vi "AuMT8852B VI Tree.vi"   [LabVIEW 2017]
doc: "This is the instrument driver for the MT8852B. The VI Tree displays all the user-callable VIs of the instrument driver in an organized table."
panel:
  # "SEE DIAGRAM\nFOR VI TREE."
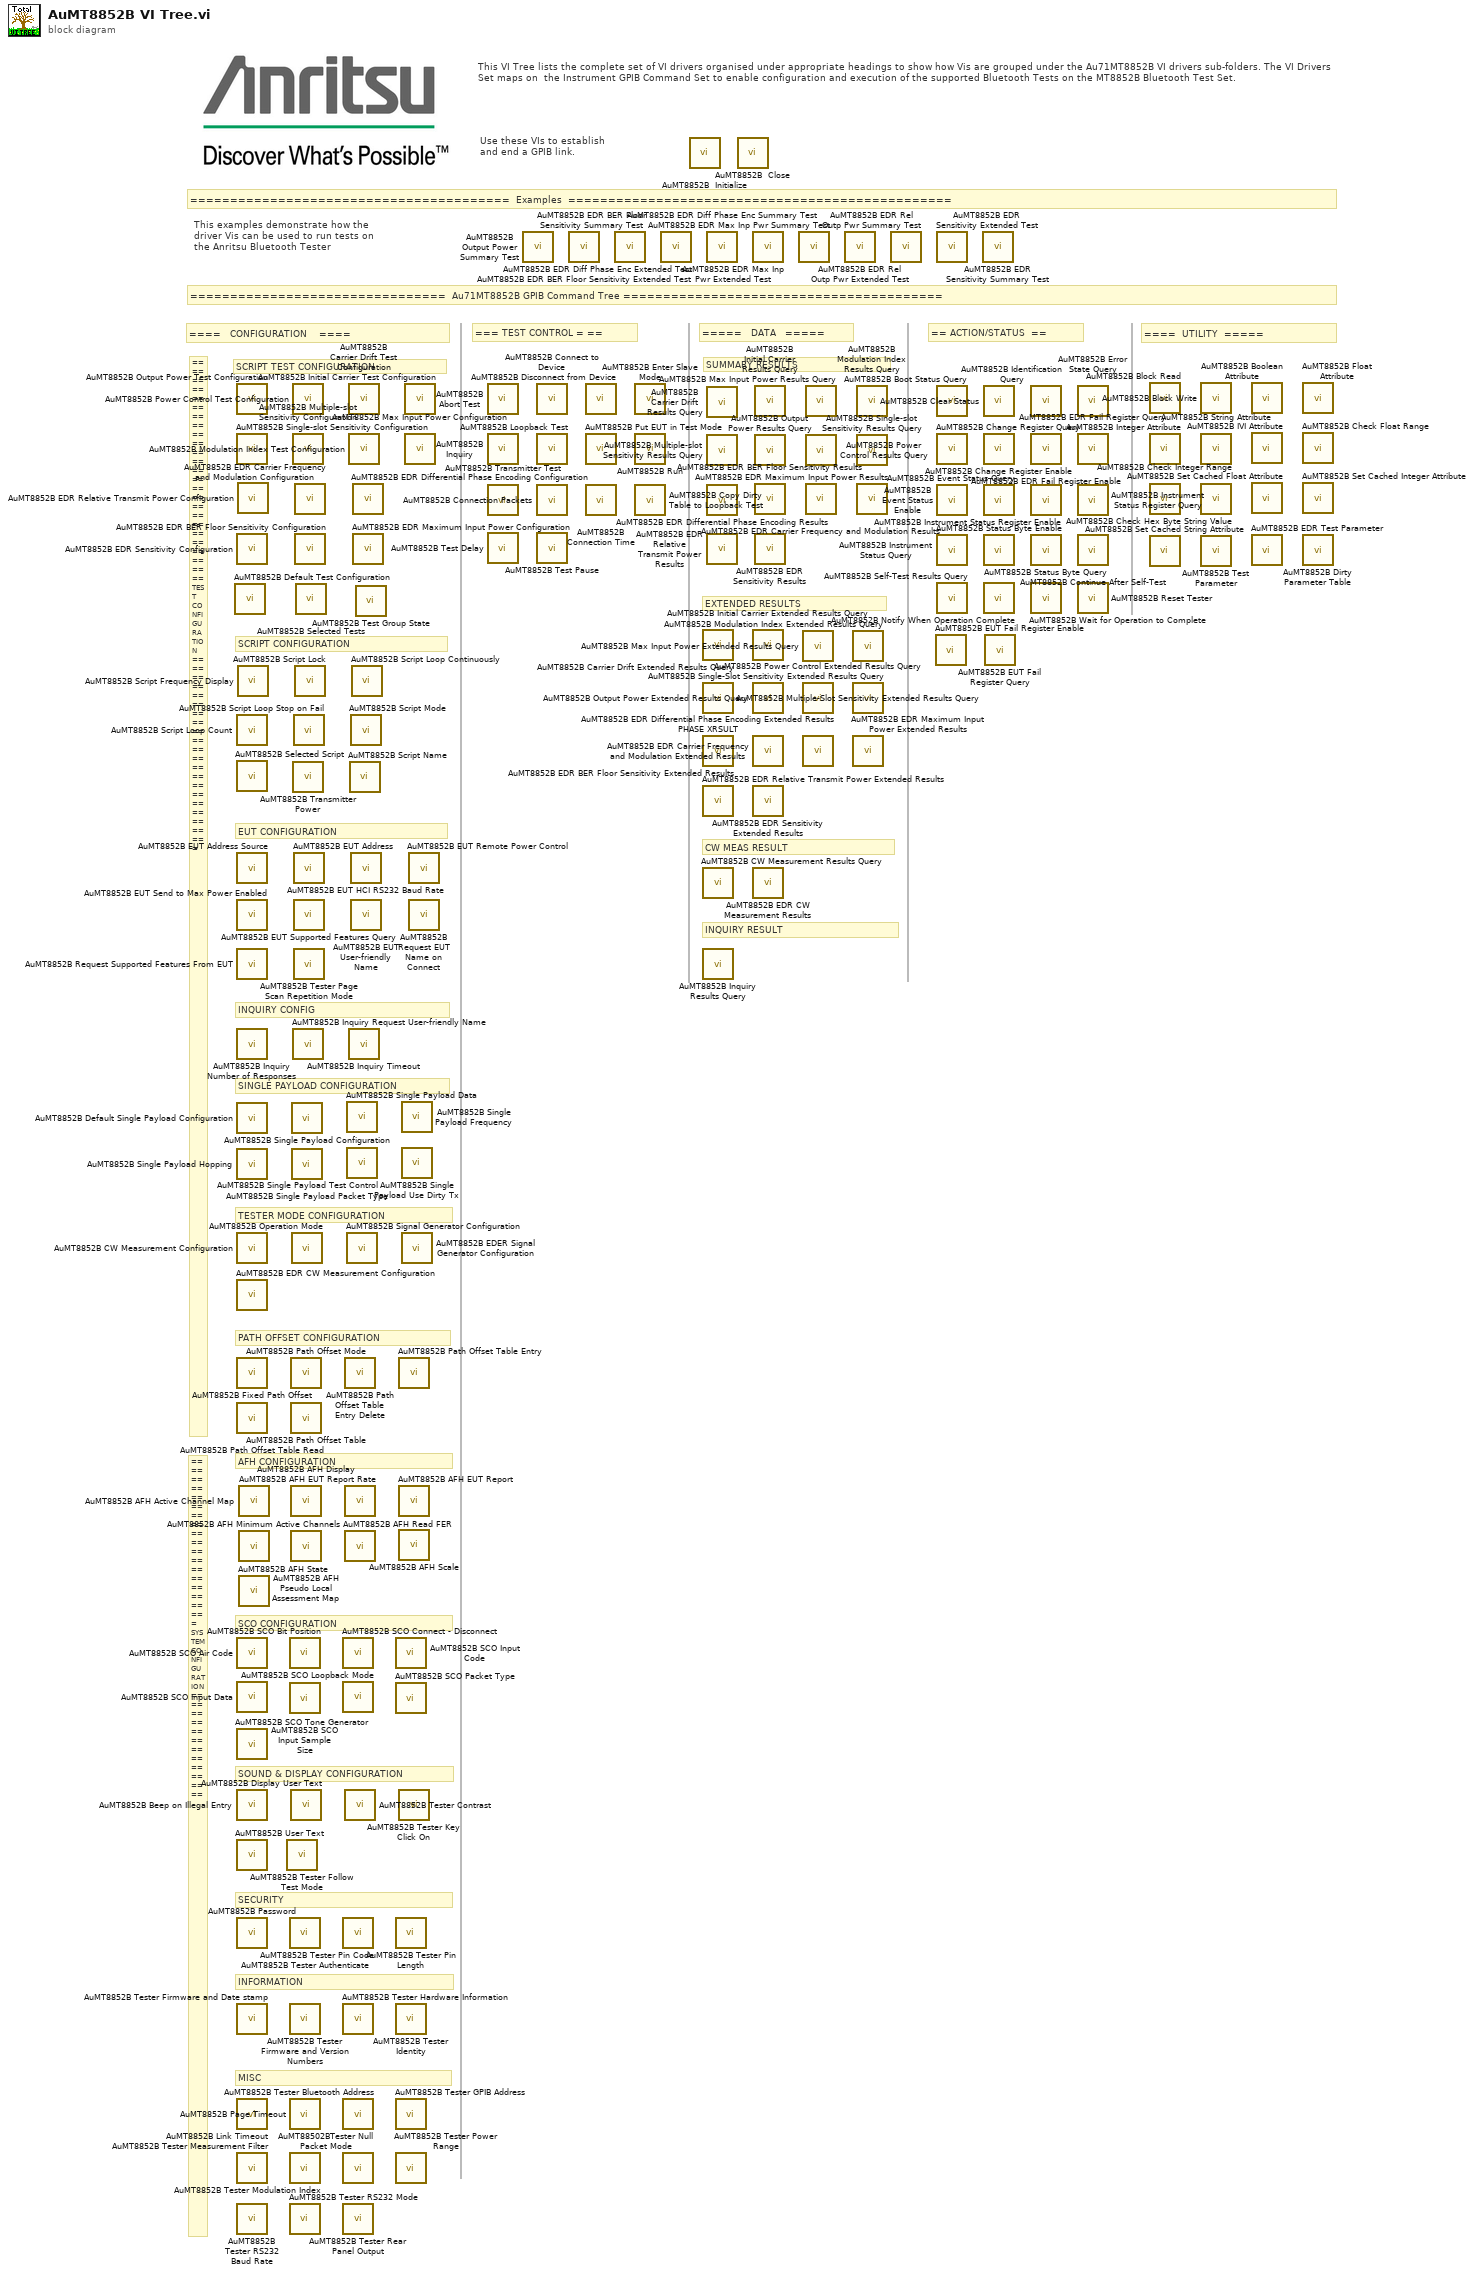
[diagram p0: block diagram]
diagram:
  # "This examples demonstrate how the \ndriver Vis can be used to run tests on \nthe Anritsu Bluetooth Tester"
  # "========================================  Examples  ================================================"
  # "=== TEST CONTROL = =="
  # "SCRIPT CONFIGURATION"
  # "===================================== SYSTEM CONFIGURATION ========================"
  # "INQUIRY RESULT"
  # "CW MEAS RESULT"
  # "EXTENDED RESULTS"
  # "SUMMARY RESULTS"
  # "MISC"
  # "INFORMATION"
  # "SECURITY"
  # "SOUND & DISPLAY CONFIGURATION"
  # "SCO CONFIGURATION"
  # "AFH CONFIGURATION"
  # "INQUIRY CONFIG"
  # "TESTER MODE CONFIGURATION"
  # "PATH OFFSET CONFIGURATION"
  # "EUT CONFIGURATION"
  # "SCRIPT TEST CONFIGURATION"
  # "SINGLE PAYLOAD CONFIGURATION"
  # "================================================== TEST CONFIGURATION ==========================================="
  # "====  UTILITY  ====="
  # "== ACTION/STATUS  =="
  # "=====   DATA   ====="
  # "This VI Tree lists the complete set of VI drivers organised under appropriate headings to show how Vis are grouped under the Au71MT8852B VI drivers sub-folders. The VI Drivers Set maps on  the Instrument GPIB Command Set to enable configuration and execution of the supported Bluetooth Tests on the MT8852B Bluetooth Test Set."
  # "Use these VIs to establish \nand end a GPIB link."
  # "====   CONFIGURATION    ===="
  # "================================  Au71MT8852B GPIB Command Tree ========================================"
  n1 = call <instrlib>:"AuMT8852B Default Test Configuration.vi"() -> ()  [unwired: 9 in, 3 out]
  n2 = call <instrlib>:"AuMT8852B Output Power Test Configuration.vi"() -> ()  [unwired: 8 in, 4 out]
  n3 = call <instrlib>:"AuMT8852B Single-slot Sensitivity Configuration.vi"() -> ()  [unwired: 8 in, 4 out]
  n4 = call <instrlib>:"AuMT8852B EDR Sensitivity Configuration.vi"() -> ()  [unwired: 8 in, 4 out]
  n5 = call <instrlib>:"AuMT8852B Script Loop Count.vi"() -> ()  [unwired: 8 in, 4 out]
  n6 = call <instrlib>:"AuMT8852B Selected Script.vi"() -> ()  [unwired: 8 in, 4 out]
  n7 = call <instrlib>:"AuMT8852B EUT Address Source.vi"() -> ()  [unwired: 8 in, 4 out]
  n8 = call <instrlib>:"AuMT8852B EUT Send to Max Power Enabled.vi"() -> ()  [unwired: 8 in, 4 out]
  n9 = call <instrlib>:"AuMT8852B Request Supported Features From EUT.vi"() -> ()  [unwired: 9 in, 3 out]
  n10 = call <instrlib>:"AuMT8852B Inquiry Number of Responses.vi"() -> ()  [unwired: 8 in, 4 out]
  n11 = call <instrlib>:"AuMT8852B Default Single Payload Configuration.vi"() -> ()  [unwired: 9 in, 3 out]
  n12 = call <instrlib>:"AuMT8852B Single Payload Hopping.vi"() -> ()  [unwired: 8 in, 4 out]
  n13 = call <instrlib>:"AuMT8852B CW Measurement Configuration.vi"() -> ()  [unwired: 6 in, 6 out]
  n14 = call <instrlib>:"AuMT8852B EDR CW Measurement Configuration.vi"() -> ()  [unwired: 8 in, 4 out]
  n15 = call <instrlib>:"AuMT8852B Fixed Path Offset.vi"() -> ()  [unwired: 8 in, 4 out]
  n16 = call <instrlib>:"AuMT8852B Path Offset Table Read.vi"() -> ()  [unwired: 8 in, 4 out]
  n17 = call <instrlib>:"AuMT8852B SCO Air Code.vi"() -> ()  [unwired: 8 in, 4 out]
  n18 = call <instrlib>:"AuMT8852B SCO Input Data.vi"() -> ()  [unwired: 8 in, 4 out]
  n19 = call <instrlib>:"AuMT8852B SCO Tone Generator.vi"() -> ()  [unwired: 8 in, 4 out]
  n20 = call <instrlib>:"AuMT8852B Beep on Illegal Entry.vi"() -> ()  [unwired: 8 in, 4 out]
  n21 = call <instrlib>:"AuMT8852B User Text.vi"() -> ()  [unwired: 8 in, 4 out]
  n22 = call <instrlib>:"AuMT8852B Password.vi"() -> ()  [unwired: 9 in, 3 out]
  n23 = call <instrlib>:"AuMT8852B Tester Firmware and Date stamp.vi"() -> ()  [unwired: 8 in, 4 out]
  n24 = call <instrlib>:"AuMT8852B Link Timeout.vi"() -> ()  [unwired: 8 in, 4 out]
  n25 = call <instrlib>:"AuMT8852B Tester Measurement Filter.vi"() -> ()  [unwired: 8 in, 4 out]
  n26 = call <instrlib>:"AuMT8852B Tester RS232 Baud Rate.vi"() -> ()  [unwired: 8 in, 4 out]
  n27 = call <instrlib>:"AuMT8852B EDR Relative Transmit Power Configuration.vi"() -> ()  [unwired: 8 in, 4 out]
  n28 = call <instrlib>:"AuMT8852B Script Frequency Display.vi"() -> ()  [unwired: 8 in, 4 out]
  n29 = call <instrlib>:"AuMT8852B AFH Active Channel Map.vi"() -> ()  [unwired: 7 in, 5 out]
  n30 = call <instrlib>:"AuMT8852B AFH Minimum Active Channels.vi"() -> ()  [unwired: 8 in, 4 out]
  n31 = call <instrlib>:"AuMT8852B AFH State.vi"() -> ()  [unwired: 8 in, 4 out]
  n32 = call <instrlib>:"AuMT8852B Tester Follow Test Mode.vi"() -> ()  [unwired: 8 in, 4 out]
  n33 = call <instrlib>:"AuMT8852B SCO Bit Position.vi"() -> ()  [unwired: 8 in, 4 out]
  n34 = call <instrlib>:"AuMT8852B SCO Input Sample Size.vi"() -> ()  [unwired: 8 in, 4 out]
  n35 = call <instrlib>:"AuMT8852B Tester Authenticate.vi"() -> ()  [unwired: 8 in, 4 out]
  n36 = call <instrlib>:"AuMT8852B Tester Firmware and Version Numbers.vi"() -> ()  [unwired: 8 in, 4 out]
  n37 = call <instrlib>:"AuMT8852B Page Timeout.vi"() -> ()  [unwired: 8 in, 4 out]
  n38 = call <instrlib>:"AuMT8852B Tester Modulation Index.vi"() -> ()  [unwired: 8 in, 4 out]
  n39 = call <instrlib>:"AuMT8852B Tester RS232 Mode.vi"() -> ()  [unwired: 8 in, 4 out]
  n40 = call <instrlib>:"AuMT8852B Path Offset Mode.vi"() -> ()  [unwired: 8 in, 4 out]
  n41 = call <instrlib>:"AuMT8852B Path Offset Table.vi"() -> ()  [unwired: 8 in, 4 out]
  n42 = call <instrlib>:"AuMT8852B AFH Display.vi"() -> ()  [unwired: 8 in, 4 out]
  n43 = call <instrlib>:"AuMT8852B AFH Pseudo Local Assessment Map.vi"() -> ()  [unwired: 9 in, 3 out]
  n44 = call <instrlib>:"AuMT8852B Display User Text.vi"() -> ()  [unwired: 8 in, 4 out]
  n45 = call <instrlib>:"AuMT8852B Single Payload Configuration.vi"() -> ()  [unwired: 8 in, 4 out]
  n46 = call <instrlib>:"AuMT8852B Single Payload Packet Type.vi"() -> ()  [unwired: 8 in, 4 out]
  n47 = call <instrlib>:"AuMT8852B Operation Mode.vi"() -> ()  [unwired: 8 in, 4 out]
  n48 = call <instrlib>:"AuMT8852B Power Control Test Configuration.vi"() -> ()  [unwired: 8 in, 4 out]
  n49 = call <instrlib>:"AuMT8852B Multiple-slot Sensitivity Configuration.vi"() -> ()  [unwired: 8 in, 4 out]
  n50 = call <instrlib>:"AuMT8852B Transmitter Power.vi"() -> ()  [unwired: 8 in, 4 out]
  n51 = call <instrlib>:"AuMT8852B Inquiry Request User-friendly Name.vi"() -> ()  [unwired: 8 in, 4 out]
  n52 = call <instrlib>:"AuMT8852B Script Loop Stop on Fail.vi"() -> ()  [unwired: 8 in, 4 out]
  n53 = call <instrlib>:"AuMT8852B EUT Address.vi"() -> ()  [unwired: 8 in, 4 out]
  n54 = call <instrlib>:"AuMT8852B EUT Supported Features Query.vi"() -> ()  [unwired: 8 in, 4 out]
  n55 = call <instrlib>:"AuMT8852B Tester Page Scan Repetition Mode.vi"() -> ()  [unwired: 8 in, 4 out]
  n56 = call <instrlib>:"AuMT8852B EDR Carrier Frequency and Modulation Configuration.vi"() -> ()  [unwired: 8 in, 4 out]
  n57 = call <instrlib>:"AuMT8852B EDR BER Floor Sensitivity Configuration.vi"() -> ()  [unwired: 8 in, 4 out]
  n58 = call <instrlib>:"AuMT8852B Script Lock.vi"() -> ()  [unwired: 8 in, 4 out]
  n59 = call <instrlib>:"AuMT8852B Selected Tests.vi"() -> ()  [unwired: 8 in, 4 out]
  n60 = call <instrlib>:"AuMT8852B SCO Connect - Disconnect.vi"() -> ()  [unwired: 9 in, 3 out]
  n61 = call <instrlib>:"AuMT8852B SCO Loopback Mode.vi"() -> ()  [unwired: 8 in, 4 out]
  n62 = call <instrlib>:"AuMT8852B Tester Pin Code.vi"() -> ()  [unwired: 8 in, 4 out]
  n63 = call <instrlib>:"AuMT8852B Tester Hardware Information.vi"() -> ()  [unwired: 8 in, 4 out]
  n64 = call <instrlib>:"AuMT8852B Tester Bluetooth Address.vi"() -> ()  [unwired: 8 in, 4 out]
  n65 = call <instrlib>:"AuMT88502BTester Null Packet Mode.vi"() -> ()  [unwired: 8 in, 4 out]
  n66 = call <instrlib>:"AuMT8852B Tester Rear Panel Output.vi"() -> ()  [unwired: 8 in, 4 out]
  n67 = call <instrlib>:"AuMT8852B Path Offset Table Entry Delete.vi"() -> ()  [unwired: 9 in, 3 out]
  n68 = call <instrlib>:"AuMT8852B AFH EUT Report Rate.vi"() -> ()  [unwired: 8 in, 4 out]
  n69 = call <instrlib>:"AuMT8852B AFH Read FER.vi"() -> ()  [unwired: 8 in, 4 out]
  n70 = call <instrlib>:"AuMT8852B Tester Contrast.vi"() -> ()  [unwired: 8 in, 4 out]
  n71 = call <instrlib>:"AuMT8852B Single Payload Data.vi"() -> ()  [unwired: 8 in, 4 out]
  n72 = call <instrlib>:"AuMT8852B Single Payload Test Control.vi"() -> ()  [unwired: 8 in, 4 out]
  n73 = call <instrlib>:"AuMT8852B Signal Generator Configuration.vi"() -> ()  [unwired: 8 in, 4 out]
  n74 = call <instrlib>:"AuMT8852B Carrier Drift Test Configuration.vi"() -> ()  [unwired: 8 in, 4 out]
  n75 = call <instrlib>:"AuMT8852B Modulation Index Test Configuration.vi"() -> ()  [unwired: 8 in, 4 out]
  n76 = call <instrlib>:"AuMT8852B Inquiry Timeout.vi"() -> ()  [unwired: 8 in, 4 out]
  n77 = call <instrlib>:"AuMT8852B Script Name.vi"() -> ()  [unwired: 8 in, 4 out]
  n78 = call <instrlib>:"AuMT8852B Script Mode.vi"() -> ()  [unwired: 8 in, 4 out]
  n79 = call <instrlib>:"AuMT8852B EUT HCI RS232 Baud Rate.vi"() -> ()  [unwired: 8 in, 4 out]
  n80 = call <instrlib>:"AuMT8852B EUT User-friendly Name.vi"() -> ()  [unwired: 8 in, 4 out]
  n81 = call <instrlib>:"AuMT8852B Script Loop Continuously.vi"() -> ()  [unwired: 8 in, 4 out]
  n82 = call <instrlib>:"AuMT8852B EDR Differential Phase Encoding Configuration.vi"() -> ()  [unwired: 8 in, 4 out]
  n83 = call <instrlib>:"AuMT8852B EDR Maximum Input Power Configuration.vi"() -> ()  [unwired: 8 in, 4 out]
  n84 = call <instrlib>:"AuMT8852B Test Group State.vi"() -> ()  [unwired: 7 in, 5 out]
  n85 = call <instrlib>:"AuMT8852B SCO Input Code.vi"() -> ()  [unwired: 8 in, 4 out]
  n86 = call <instrlib>:"AuMT8852B SCO Packet Type.vi"() -> ()  [unwired: 8 in, 4 out]
  n87 = call <instrlib>:"AuMT8852B Tester Pin Length.vi"() -> ()  [unwired: 8 in, 4 out]
  n88 = call <instrlib>:"AuMT8852B Tester Identity.vi"() -> ()  [unwired: 8 in, 4 out]
  n89 = call <instrlib>:"AuMT8852B Tester GPIB Address.vi"() -> ()  [unwired: 8 in, 4 out]
  n90 = call <instrlib>:"AuMT8852B Tester Power Range.vi"() -> ()  [unwired: 8 in, 4 out]
  n91 = call <instrlib>:"AuMT8852B Path Offset Table Entry.vi"() -> ()  [unwired: 8 in, 4 out]
  n92 = call <instrlib>:"AuMT8852B AFH EUT Report.vi"() -> ()  [unwired: 8 in, 4 out]
  n93 = call <instrlib>:"AuMT8852B AFH Scale.vi"() -> ()  [unwired: 8 in, 4 out]
  n94 = call <instrlib>:"AuMT8852B Tester Key Click On.vi"() -> ()  [unwired: 8 in, 4 out]
  n95 = call <instrlib>:"AuMT8852B Single Payload Frequency.vi"() -> ()  [unwired: 8 in, 4 out]
  n96 = call <instrlib>:"AuMT8852B Single Payload Use Dirty Tx.vi"() -> ()  [unwired: 8 in, 4 out]
  n97 = call <instrlib>:"AuMT8852B EDER Signal Generator Configuration.vi"() -> ()  [unwired: 8 in, 4 out]
  n98 = call <instrlib>:"AuMT8852B Initial Carrier Test Configuration.vi"() -> ()  [unwired: 8 in, 4 out]
  n99 = call <instrlib>:"AuMT8852B Max Input Power Configuration.vi"() -> ()  [unwired: 8 in, 4 out]
  n100 = call <instrlib>:"AuMT8852B EUT Remote Power Control.vi"() -> ()  [unwired: 9 in, 3 out]
  n101 = call <instrlib>:"AuMT8852B Request EUT Name on Connect.vi"() -> ()  [unwired: 8 in, 4 out]
  n102 = call <instrlib>:"AuMT8852B Abort Test.vi"() -> ()  [unwired: 9 in, 3 out]
  n103 = call <instrlib>:"AuMT8852B Inquiry.vi"() -> ()  [unwired: 9 in, 3 out]
  n104 = call <instrlib>:"AuMT8852B Transmitter Test.vi"() -> ()  [unwired: 9 in, 3 out]
  n105 = call <instrlib>:"AuMT8852B Test Delay.vi"() -> ()  [unwired: 8 in, 4 out]
  n106 = call <instrlib>:"AuMT8852B Output Power Summary Test.vi"() -> ()  [unwired: 1 in]
  n107 = call <instrlib>:"AuMT8852B Connect to Device.vi"() -> ()  [unwired: 9 in, 3 out]
  n108 = call <instrlib>:"AuMT8852B Loopback Test.vi"() -> ()  [unwired: 9 in, 3 out]
  n109 = call <instrlib>:"AuMT8852B Connection Packets.vi"() -> ()  [unwired: 8 in, 4 out]
  n110 = call <instrlib>:"AuMT8852B Test Pause.vi"() -> ()  [unwired: 8 in, 4 out]
  n111 = call <instrlib>:"AuMT8852B EDR BER Floor Sensitivity Extended Test.vi"() -> ()  [unwired: 1 in]
  n112 = call <instrlib>:"AuMT8852B Disconnect from Device.vi"() -> ()  [unwired: 9 in, 3 out]
  n113 = call <instrlib>:"AuMT8852B Put EUT in Test Mode.vi"() -> ()  [unwired: 9 in, 3 out]
  n114 = call <instrlib>:"AuMT8852B Connection Time.vi"() -> ()  [unwired: 8 in, 4 out]
  n115 = call <instrlib>:"AuMT8852B EDR BER Floor Sensitivity Summary Test.vi"() -> ()  [unwired: 1 in]
  n116 = call <instrlib>:"AuMT8852B Enter Slave Mode.vi"() -> ()  [unwired: 9 in, 3 out]
  n117 = call <instrlib>:"AuMT8852B Run.vi"() -> ()  [unwired: 9 in, 3 out]
  n118 = call <instrlib>:"AuMT8852B Copy Dirty Table to Loopback Test.vi"() -> ()  [unwired: 9 in, 3 out]
  n119 = call <instrlib>:"AuMT8852B EDR Diff Phase Enc Extended Test.vi"() -> ()  [unwired: 1 in]
  n120 = call <instrlib>:"AuMT8852B  Initialize.vi"() -> ()  [unwired: 10 in, 2 out]
  n121 = call <instrlib>:"AuMT8852B Carrier Drift Extended Results Query.vi"() -> ()  [unwired: 8 in, 4 out]
  n122 = call <instrlib>:"AuMT8852B Multiple-Slot Sensitivity Extended Results Query.vi"() -> ()  [unwired: 8 in, 4 out]
  n123 = call <instrlib>:"AuMT8852B EDR BER Floor Sensitivity Extended Results.vi"() -> ()  [unwired: 8 in, 4 out]
  n124 = call <instrlib>:"AuMT8852B EDR Relative Transmit Power Extended Results.vi"() -> ()  [unwired: 8 in, 4 out]
  n125 = call <instrlib>:"AuMT8852B CW Measurement Results Query.vi"() -> ()  [unwired: 8 in, 4 out]
  n126 = call <instrlib>:"AuMT8852B Inquiry Results Query.vi"() -> ()  [unwired: 7 in, 5 out]
  n127 = call <instrlib>:"AuMT8852B EDR Diff Phase Enc Summary Test.vi"() -> ()  [unwired: 1 in]
  n128 = call <instrlib>:"AuMT8852B Carrier Drift Results Query.vi"() -> ()  [unwired: 8 in, 4 out]
  n129 = call <instrlib>:"AuMT8852B Multiple-slot Sensitivity Results Query.vi"() -> ()  [unwired: 8 in, 4 out]
  n130 = call <instrlib>:"AuMT8852B EDR Differential Phase Encoding Results.vi"() -> ()  [unwired: 8 in, 4 out]
  n131 = call <instrlib>:"AuMT8852B EDR Relative Transmit Power Results.vi"() -> ()  [unwired: 8 in, 4 out]
  n132 = call <instrlib>:"AuMT8852B  Close.vi"() -> ()  [unwired: 10 in, 2 out]
  n133 = call <instrlib>:"AuMT8852B EDR Max Inp Pwr Extended Test.vi"() -> ()  [unwired: 1 in]
  n134 = call <instrlib>:"AuMT8852B Initial Carrier Extended Results Query.vi"() -> ()  [unwired: 8 in, 4 out]
  n135 = call <instrlib>:"AuMT8852B Output Power Extended Results Query.vi"() -> ()  [unwired: 8 in, 4 out]
  n136 = call <instrlib>:"AuMT8852B EDR Carrier Frequency and Modulation Extended Results.vi"() -> ()  [unwired: 8 in, 4 out]
  n137 = call <instrlib>:"AuMT8852B EDR Sensitivity Extended Results.vi"() -> ()  [unwired: 8 in, 4 out]
  n138 = call <instrlib>:"AuMT8852B EDR CW Measurement Results.vi"() -> ()  [unwired: 8 in, 4 out]
  n139 = call <instrlib>:"AuMT8852B Initial Carrier Results Query.vi"() -> ()  [unwired: 8 in, 4 out]
  n140 = call <instrlib>:"AuMT8852B Output Power Results Query.vi"() -> ()  [unwired: 8 in, 4 out]
  n141 = call <instrlib>:"AuMT8852B EDR BER Floor Sensitivity Results.vi"() -> ()  [unwired: 8 in, 4 out]
  n142 = call <instrlib>:"AuMT8852B EDR Sensitivity Results.vi"() -> ()  [unwired: 8 in, 4 out]
  n143 = call <instrlib>:"AuMT8852B EDR Max Inp Pwr Summary Test.vi"() -> ()  [unwired: 1 in]
  n144 = call <instrlib>:"AuMT8852B Max Input Power Extended Results Query.vi"() -> ()  [unwired: 8 in, 4 out]
  n145 = call <instrlib>:"AuMT8852B Power Control Extended Results Query.vi"() -> ()  [unwired: 8 in, 4 out]
  n146 = call <instrlib>:"AuMT8852B EDR Differential Phase Encoding Extended Results PHASE XRSULT.vi"() -> ()  [unwired: 8 in, 4 out]
  n147 = call <instrlib>:"AuMT8852B Max Input Power Results Query.vi"() -> ()  [unwired: 8 in, 4 out]
  n148 = call <instrlib>:"AuMT8852B Power Control Results Query.vi"() -> ()  [unwired: 8 in, 4 out]
  n149 = call <instrlib>:"AuMT8852B EDR Carrier Frequency and Modulation Results.vi"() -> ()  [unwired: 8 in, 4 out]
  n150 = call <instrlib>:"AuMT8852B EDR Rel Outp Pwr Extended Test.vi"() -> ()  [unwired: 1 in]
  n151 = call <instrlib>:"AuMT8852B Modulation Index Extended Results Query.vi"() -> ()  [unwired: 8 in, 4 out]
  n152 = call <instrlib>:"AuMT8852B Single-Slot Sensitivity Extended Results Query.vi"() -> ()  [unwired: 8 in, 4 out]
  n153 = call <instrlib>:"AuMT8852B EDR Maximum Input Power Extended Results.vi"() -> ()  [unwired: 8 in, 4 out]
  n154 = call <instrlib>:"AuMT8852B Modulation Index Results Query.vi"() -> ()  [unwired: 8 in, 4 out]
  n155 = call <instrlib>:"AuMT8852B Single-slot Sensitivity Results Query.vi"() -> ()  [unwired: 8 in, 4 out]
  n156 = call <instrlib>:"AuMT8852B EDR Maximum Input Power Results.vi"() -> ()  [unwired: 8 in, 4 out]
  n157 = call <instrlib>:"AuMT8852B EDR Rel Outp Pwr Summary Test.vi"() -> ()  [unwired: 1 in]
  n158 = call <instrlib>:"AuMT8852B EUT Fail Register Enable.vi"() -> ()  [unwired: 7 in, 5 out]
  n159 = call <instrlib>:"AuMT8852B EDR Sensitivity Extended Test.vi"() -> ()  [unwired: 1 in]
  n160 = call <instrlib>:"AuMT8852B Boot Status Query.vi"() -> ()  [unwired: 8 in, 4 out]
  n161 = call <instrlib>:"AuMT8852B Change Register Query.vi"() -> ()  [unwired: 7 in, 5 out]
  n162 = call <instrlib>:"AuMT8852B Event Status Enable.vi"() -> ()  [unwired: 7 in, 5 out]
  n163 = call <instrlib>:"AuMT8852B Instrument Status Query.vi"() -> ()  [unwired: 8 in, 4 out]
  n164 = call <instrlib>:"AuMT8852B Self-Test Results Query.vi"() -> ()  [unwired: 8 in, 4 out]
  n165 = call <instrlib>:"AuMT8852B EDR Sensitivity Summary Test.vi"() -> ()  [unwired: 1 in]
  n166 = call <instrlib>:"AuMT8852B Clear Status.vi"() -> ()  [unwired: 9 in, 3 out]
  n167 = call <instrlib>:"AuMT8852B Change Register Enable.vi"() -> ()  [unwired: 8 in, 4 out]
  n168 = call <instrlib>:"AuMT8852B Event Status Query.vi"() -> ()  [unwired: 7 in, 5 out]
  n169 = call <instrlib>:"AuMT8852B Status Byte Enable.vi"() -> ()  [unwired: 7 in, 5 out]
  n170 = call <instrlib>:"AuMT8852B Notify When Operation Complete.vi"() -> ()  [unwired: 9 in, 3 out]
  n171 = call <instrlib>:"AuMT8852B EUT Fail Register Query.vi"() -> ()  [unwired: 7 in, 5 out]
  n172 = call <instrlib>:"AuMT8852B Identification Query.vi"() -> ()  [unwired: 8 in, 4 out]
  n173 = call <instrlib>:"AuMT8852B EDR Fail Register Enable.vi"() -> ()  [unwired: 7 in, 5 out]
  n174 = call <instrlib>:"AuMT8852B Instrument Status Register Enable.vi"() -> ()  [unwired: 7 in, 5 out]
  n175 = call <instrlib>:"AuMT8852B Status Byte Query.vi"() -> ()  [unwired: 7 in, 5 out]
  n176 = call <instrlib>:"AuMT8852B Wait for Operation to Complete.vi"() -> ()  [unwired: 9 in, 3 out]
  n177 = call <instrlib>:"AuMT8852B Error State Query.vi"() -> ()  [unwired: 8 in, 4 out]
  n178 = call <instrlib>:"AuMT8852B EDR Fail Register Query.vi"() -> ()  [unwired: 7 in, 5 out]
  n179 = call <instrlib>:"AuMT8852B Instrument Status Register Query.vi"() -> ()  [unwired: 7 in, 5 out]
  n180 = call <instrlib>:"AuMT8852B Continue After Self-Test.vi"() -> ()  [unwired: 9 in, 3 out]
  n181 = call <instrlib>:"AuMT8852B Reset Tester.vi"() -> ()  [unwired: 9 in, 3 out]
  n182 = call <instrlib>:"AuMT8852B Block Read.vi"() -> ()  [unwired: 9 in, 3 out]
  n183 = call <instrlib>:"AuMT8852B Integer Attribute.vi"() -> ()  [unwired: 8 in, 4 out]
  n184 = call <instrlib>:"AuMT8852B Check Integer Range.vi"() -> ()  [unwired: 10 in, 2 out]
  n185 = call <instrlib>:"AuMT8852B Set Cached String Attribute.vi"() -> ()  [unwired: 10 in, 2 out]
  n186 = call <instrlib>:"AuMT8852B Block Write.vi"() -> ()  [unwired: 10 in, 2 out]
  n187 = call <instrlib>:"AuMT8852B String Attribute.vi"() -> ()  [unwired: 8 in, 4 out]
  n188 = call <instrlib>:"AuMT8852B Check Hex Byte String Value.vi"() -> ()  [unwired: 9 in, 3 out]
  n189 = call <instrlib>:"AuMT8852B Test Parameter.vi"() -> ()  [unwired: 16 in, 4 out]
  n190 = call <instrlib>:"AuMT8852B Boolean Attribute.vi"() -> ()  [unwired: 8 in, 4 out]
  n191 = call <instrlib>:"AuMT8852B IVI Attribute.vi"() -> ()  [unwired: 9 in, 3 out]
  n192 = call <instrlib>:"AuMT8852B Set Cached Float Attribute.vi"() -> ()  [unwired: 10 in, 2 out]
  n193 = call <instrlib>:"AuMT8852B EDR Test Parameter.vi"() -> ()  [unwired: 16 in, 4 out]
  n194 = call <instrlib>:"AuMT8852B Float Attribute.vi"() -> ()  [unwired: 8 in, 4 out]
  n195 = call <instrlib>:"AuMT8852B Check Float Range.vi"() -> ()  [unwired: 10 in, 2 out]
  n196 = call <instrlib>:"AuMT8852B Set Cached Integer Attribute.vi"() -> ()  [unwired: 10 in, 2 out]
  n197 = call <instrlib>:"AuMT8852B Dirty Parameter Table.vi"() -> ()  [unwired: 17 in, 3 out]
